vi "Win32API.vi"() -> ()   [LabVIEW 2020]
uses:
  user32.dll
panel:
  out "return type":i32
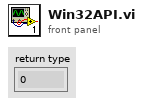
[diagram p1: front panel]
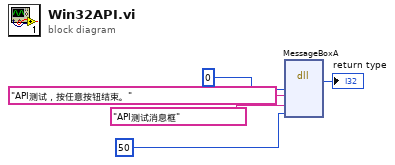
[diagram p0: block diagram]
diagram:
  n1 = dll-call lib="user32.dll" fn="MessageBoxA"("hWnd"=u32 0, "lpText"="API测试，按任意按钮结束。", "lpCaption"="API测试消息框", "uType"=50) -> ("return type"=→"return type":i32)  [unwired: 7 in, 2 out]
